vi "Select_Test_Sig_Level.vi"(11 "DeviceType":string) -> (0 "error out":errorcluster, 2 "Test_Voltage":dbl)   [LabVIEW 2020]
panel:
  in  "error in":errorcluster
  in  "Device Types":u16(ring) items=["Test Signal Level = 20mV RMS (Standard)", "Test Signal Level = 30mV RMS", "Test Signal Level = 50mV RMS", "Test Signal Level = 75mV RMS", "Test Signal Level = 100mV RMS"]
  in  "Strings []":string[](array[string])
  in  "Signal Level":string(combo)
  in  "Stop Scan":bool=TRUE
  out "Keystate":string
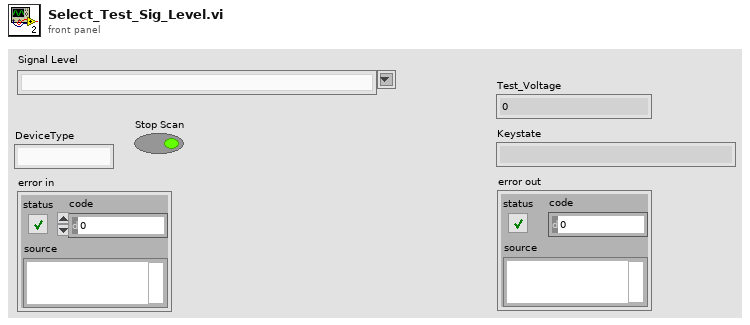
[diagram p1: front panel]
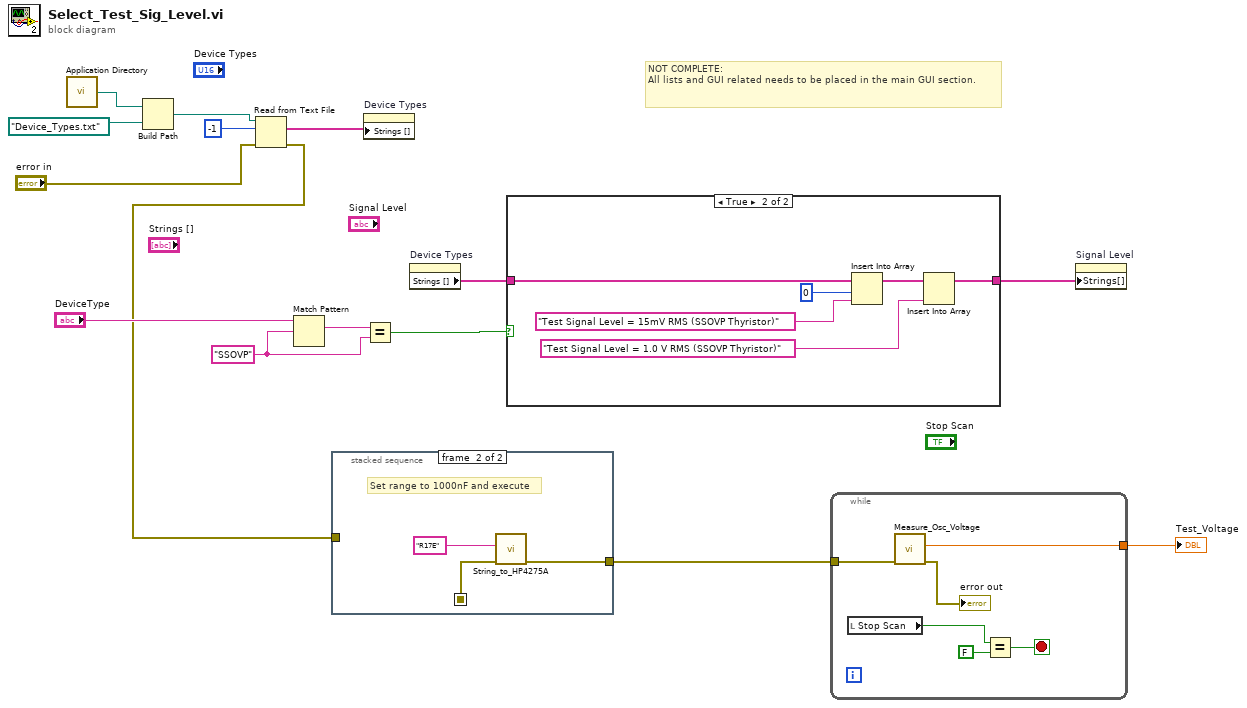
[diagram p0: block diagram]
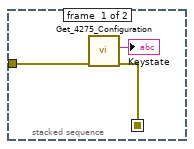
[diagram p3: hidden frame]
diagram:
  w11 = "SSOVP" ("regular expression")
  # "NOT COMPLETE:\nAll lists and GUI related needs to be placed in the main GUI section."
  n1 = call <vilib>:"Application Directory.vi"() -> ("Application Directory"=w8:path)
  n2 = Build Path(base path=w8, name or relative path=path "Device_Types.txt") -> (appended path=w4:path)
  n3 = Read from Text File(file (use dialog)=w4, count=-1, error in="error in") -> (text=w3:string[], error out=w2:errorcluster)  [unwired: 1 in, 2 out]
  n4 = Match Pattern(string="DeviceType", regular expression=w11) -> (match substring=w12:string)  [unwired: 1 in, 3 out]
  n5 = stacked-sequence {
    seq-local: [w17 _] -> [_ w20]
    tunnel: w2 -> [w18 _]
    tunnel: [_ w21] -> w15
    frame #0 {
      n6 = call "Get_4275_Configuration.vi"("error in"=w18) -> ("error out"=w17:errorcluster, "Keystate"=→"Keystate":string)  [unwired: 9 in]
    }
    frame #1 {
      # "Set range to 1000nF and execute"
      n7 = call "String_to_HP4275A.vi"("error in"=w20, "String to HP 4275A"="R17E" ("data")) -> ("error out"=w21:errorcluster)  [unwired: 9 in]
    }
  }
  n8 = property on="Device Types" class="Ring (strict)"("Strings []"=w3) -> ()  [unwired: 2 in, 2 out]
  n9 = Equal?(x=w12, y=w11) -> (x = y?=w10:bool)
  n10 = property on="Device Types" class="Ring (strict)"() -> ("Strings []"=w6:string[])  [unwired: 2 in, 2 out]
  n11 = case shown="True" w10 {
    tunnel: w6 -> [w22 w28]
    tunnel: [w22 w24] -> w14
    frame False {
    }
    frame True {
      n12 = Insert Into Array(array=w28, index=0, new element="Test Signal Level = 15mV RMS (SSOVP Thyristor)" ("new element/subarray")) -> (w25:string[])
      n13 = Insert Into Array(array=w25, new element="Test Signal Level = 1.0 V RMS (SSOVP Thyristor)" ("new element/subarray")) -> (w24:string[])  [unwired: 1 in]
    }
  }
  n14 = while {
    tunnel: w15 -> [w34]
    tunnel: [w29] -> w9
    stop <- w31 stop-if-true
    n15 = local read "Stop Scan"() -> (w30:bool)
    n16 = call "Measure_Osc_Voltage.vi"("error in"=w34) -> ("error out"=→"error out":errorcluster, "OscVoltage"=w29:dbl)  [unwired: 9 in]
    n17 = Equal?(x=w30, y=FALSE) -> (x = y?=w31:bool)
  }
  "Test_Voltage" <- w9
  n18 = property on="Signal Level" class="CmbBox"("Strings[]"=w14) -> ()  [unwired: 2 in, 2 out]
